vi "AppBar Variables.vi"() -> (1 "App Bar Height":i32=100, 2 "App Bar Peek Height":u32=24)   [LabVIEW 2012, in "Win8uiFramework.lvlib" / "MainController.lvclass"]
uses:
  MainController.lvclass
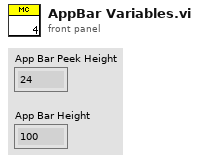
[diagram p1: front panel]
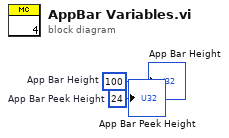
[diagram p0: block diagram]
diagram:
  w2 = u32 24  # App Bar Peek Height
  w1 = 100  # App Bar Height
  "App Bar Peek Height" <- w2
  "App Bar Height" <- w1
